vi "NetComm_CAN_CloseStreamSession.vi"(8 "error in (no error)":errorcluster, 11 "Session Handle":u32) -> (0 "error out":errorcluster)   [LabVIEW 2017]
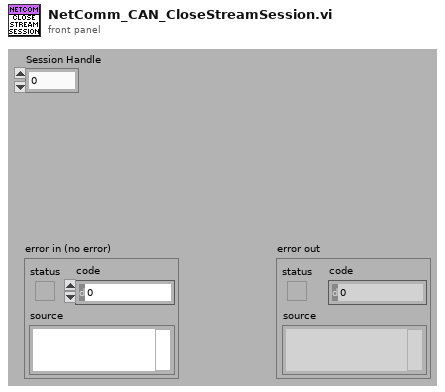
[diagram p1: front panel]
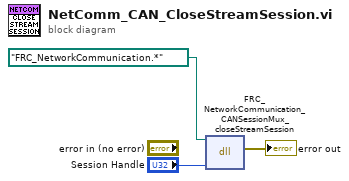
[diagram p0: block diagram]
diagram:
  n1 = dll-call lib="FRC_NetworkCommunication.*" fn="FRC_NetworkCommunication_CANSessionMux_closeStreamSession"(path in=path "FRC_NetworkCommunication.*", "sessionHandle"="Session Handle") -> (error out=→"error out":errorcluster)  [unwired: 4 in, 1 out]
